vi "Choose_USB.vi"() -> (2 "Annulé?":bool, 3 "Nom de ressource VISA en sortie":refnum<visa-resource-name>)   [LabVIEW 2014]
panel:
  in  "Bouton Annuler":bool
  in  "Bouton OK":bool
  in  "Nom de ressource VISA":refnum<visa-resource-name>
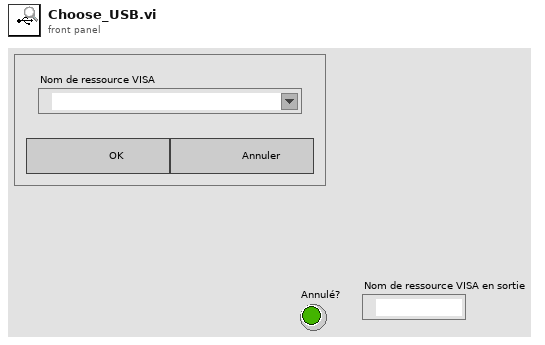
[diagram p1: front panel]
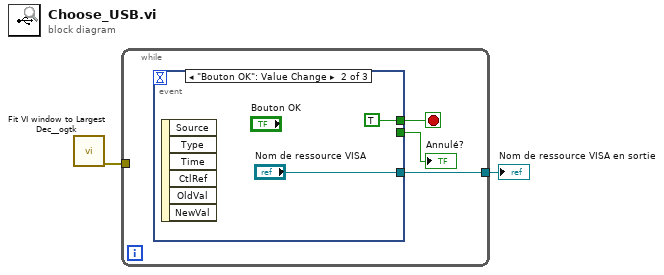
[diagram p0: block diagram]
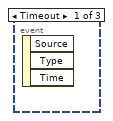
[diagram p2: hidden frame]
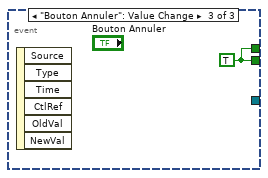
[diagram p3: hidden frame]
diagram:
  n1 = call <userlib>:"Fit VI window to Largest Dec__ogtk.vi"() -> ("error out"=w1:errorcluster)  [unwired: 6 in, 1 out]
  n2 = while {
    tunnel: [w3] -> w2
    tunnel: w1 -> [_]
    stop <- w5 stop-if-true
    n3 = event shown="[1] \"Bouton OK\": Value Change" {
      selector: _ -> [_ _ _]
      dyn-events: _ -> [_ _ _]
      timeout: _ -> [_ _ _]
      tunnel: [_ TRUE w8] -> w5
      tunnel: [_ _ w8] -> w4
      tunnel: [_ "Nom de ressource VISA" _] -> w3
      event Timeout {
        n4 = event-data() -> ()  [unwired: 1 in, 3 out]
      }
      event "Bouton OK": Value Change {
        n5 = event-data() -> ()  [unwired: 1 in, 6 out]
      }
      event "Bouton Annuler": Value Change {
        w8 = TRUE
        n6 = event-data() -> ()  [unwired: 1 in, 6 out]
      }
    }
    "Annulé?" <- w4
  }
  "Nom de ressource VISA en sortie" <- w2
